vi "Parse Entity.vi"(6 "max offset":i32, 8 "error in":errorcluster, 9 "offset (0)":i32, 10 "XML in":string) -> (0 "error out":errorcluster, 1 "offset past match":i32, 2 "element":T1, 4 "found?":bool)   [LabVIEW 2011]
uses:
  Type Defs/XML Element Table - Cluster.ctl
  Type Defs/Node Info - Cluster.ctl
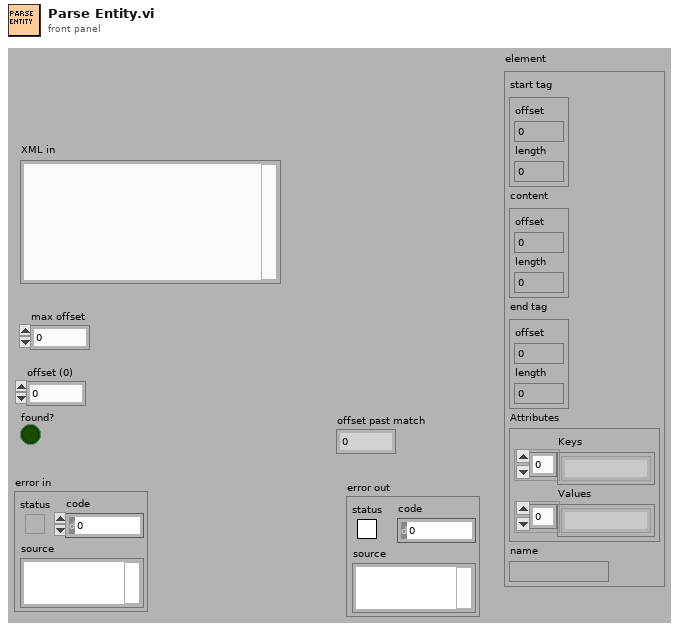
[diagram p1: front panel]
types:
  T1 = typedef "XML Element Table - Cluster.ctl" = cluster{"start tag":T2, "content":T2, "end tag":T2, "Attributes":cluster{"Keys":string[], "Values":string[]}, "name":string}
  T2 = typedef "Node Info - Cluster.ctl" = cluster{"offset":i32, "length":i32}
  T3 = cluster{"start tag":T2, "content":T2, "close tag":T2, "Attributes":cluster{"Keys":string[], "Values":string[]}, "element name":string}
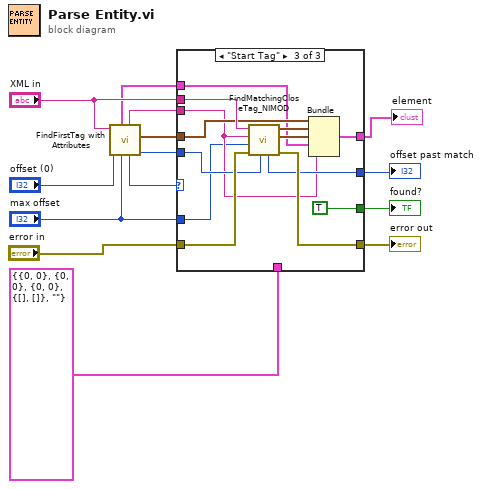
[diagram p0: block diagram]
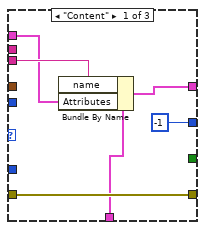
[diagram p2: hidden frame]
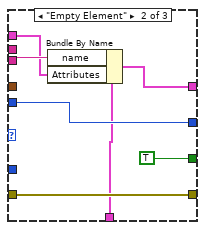
[diagram p3: hidden frame]
diagram:
  n1 = call "FindFirstTag with Attributes.vi"("max offset"="max offset", "offset (0)"="offset (0)", "XML String In"="XML in") -> ("offset past match"=w7:i32, "start tag"=w8:T2, "case"=w12:enum16{"Start Tag", "Empty Element", "Content"}, "element name"=w3:string, "Attributes"=w4:cluster{"Keys":string[], "Values":string[]})  [unwired: 4 in]
  n2 = case shown="\"Start Tag\"" w12 {
    tunnel: w3 -> [w18 w23 w30]
    tunnel: [w20 w26 w40] -> w14
    tunnel: "error in" -> [w20 w26 w39]
    tunnel: [_ TRUE ("found?") TRUE ("found?")] -> w11
    tunnel: "XML in" -> [_ _ w37]
    tunnel: w8 -> [_ _ w32]
    tunnel: w7 -> [_ w25 w36]
    tunnel: [-1 ("offset past close tag") w25 w35] -> w6
    tunnel: [w16 w22 w28] -> w5
    tunnel: w4 -> [w15 w21 w31]
    tunnel: T1 {"start tag"={"offset"=0, "length"=0}, "content"={"offset"=0, "length"=0}, "end tag"={"offset"=0, "length"=0}, "Attributes"={"Keys"=[], "Values"=[]}, "name"=""} ("element") -> [w17 w24 _]
    tunnel: "max offset" -> [_ _ w29]
    frame "Content" {
      n3 = Bundle By Name(cluster=w17, "name"=w18, "Attributes"=w15) -> (w16:T1)
    }
    frame "Empty Element" {
      n4 = Bundle By Name(cluster=w24, "name"=w23, "Attributes"=w21) -> (w22:T1)
    }
    frame "Start Tag" {
      n5 = call "FindMatchingCloseTag_NIMOD.vi"("offset (0)"=w36, "error in"=w39, "max offset"=w29, "element name"=w30, "XML string in"=w37) -> ("error out"=w40:errorcluster, "close tag"=w33:T2, "content"=w34:T2, "offset past close tag"=w35:i32)  [unwired: 3 in]
      n6 = Bundle("start tag"=w32, "content"=w34, "close tag"=w33, "Attributes"=w31, "element name"=w30) -> (w28:T3)  [unwired: 1 in]
    }
  }
  "element" <- w5
  "found?" <- w11
  "error out" <- w14
  "offset past match" <- w6
